vi "HEWH HeatUp Test Selector.vi"(4 "Standard Heat-Up (80 Gallon) Heat Pump":T1[](array[typedef]) {"Time" format="%<%H:%M:%S>t"}, 6 "Standard Heat-Up (80 Gallon)":T1[](array[typedef]) {"Time" format="%<%H:%M:%S>t"}, 7 "Standard Heat-Up (50 Gallon) Heat Pump in":T1[](array[typedef]) {"Time" format="%<%H:%M:%S>t"}, 8 "Error In":errorcluster, 9 "Heating Mode":string, 10 "Unit Type":T8, 11 "Standard Heat-Up (50 Gallon)":T1[](array[typedef]) {"Time" format="%<%H:%M:%S>t"}) -> (0 "Error Out":errorcluster, 3 "Standard Heat-Up (50 Gallon) Heat Pump out":T1[](array[typedef]) {"Time" format="%<%H:%M:%S>t"})   [LabVIEW 2016]
uses:
  Type Definitions/PRAT Test.ctl
  Utility/Save File/File Setup (Public)/Type Definition/Save File HEWH Heating Control Mode.ctl
  Draw Water Specific/Type Definitions/Terminate Draw Conditions.ctl
  Type Definitions/HEWH Start Conditions.ctl
  Draw Water Specific/Type Definitions/Check Special Condtions.ctl
  Draw Water Specific/Type Definitions/HEWH Special Condition Check.ctl
  Type Definitions/HEWH Draw Flag ENUM.ctl
  Draw Water Specific/Type Definitions/Unit Type.ctl
  Utility/Save File/File Setup.lvlib
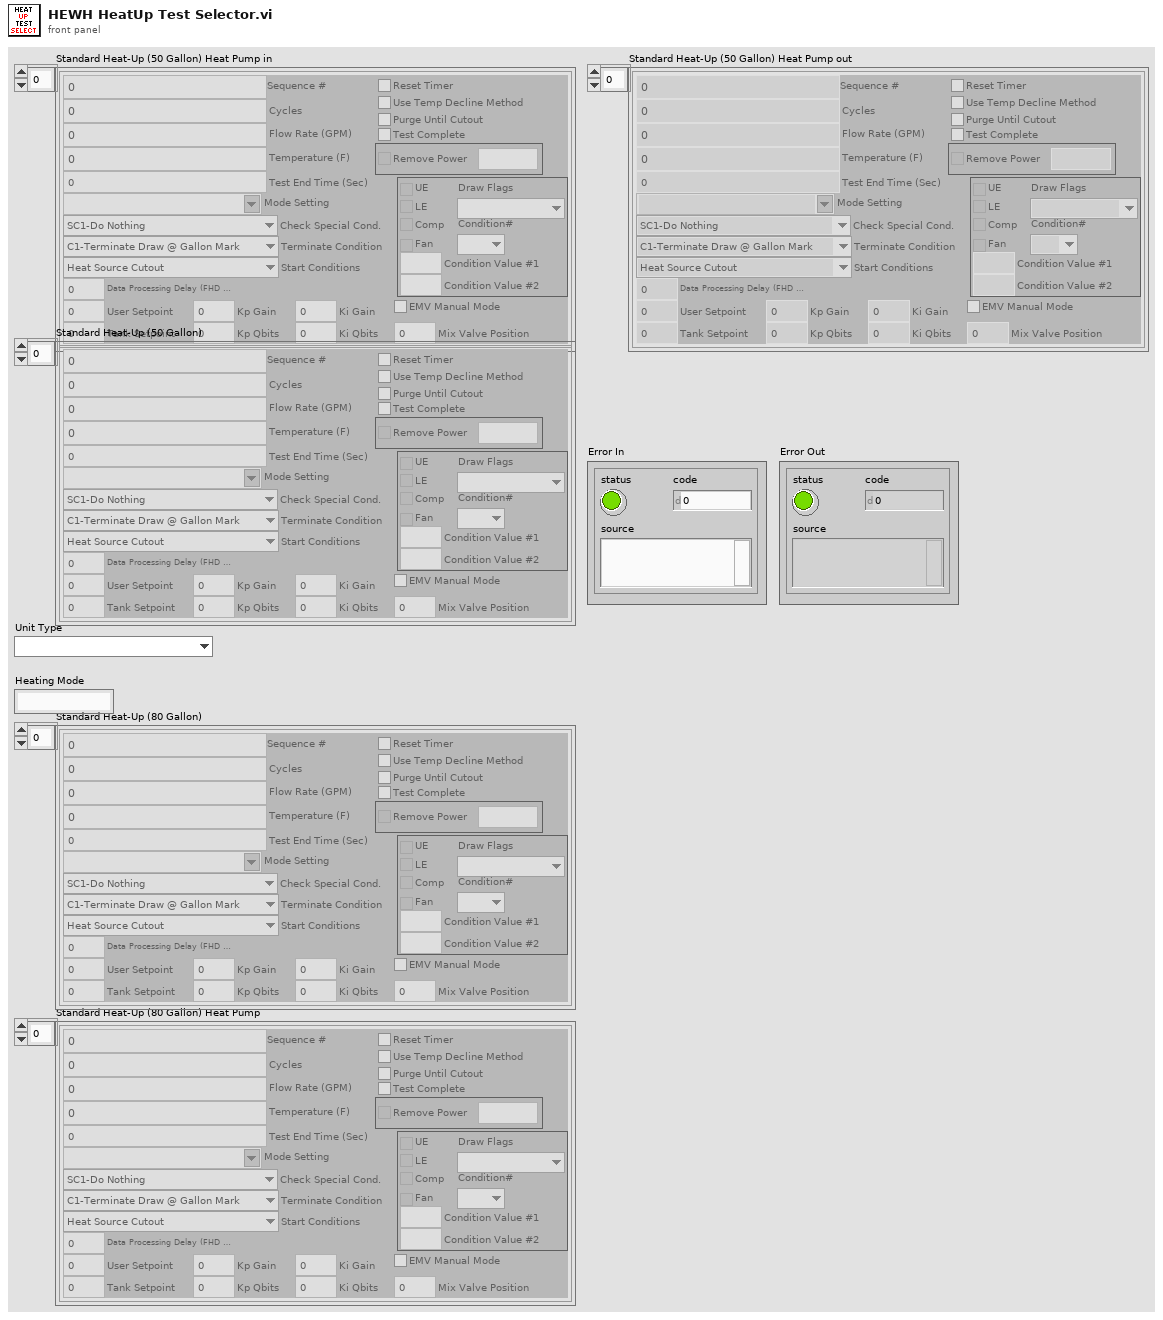
[diagram p1: front panel]
types:
  T1 = typedef "PRAT Test.ctl" = cluster{"Sequence #":dbl, "Cycles":i32, "Mode Setting":T2, "Flow Rate (GPM)":dbl, "Temperature (F)":dbl, "Reset Timer":bool, "Use Temp Decline Method":bool, "Terminate Condition":T3, "Condition Value #1":dbl, "UE":bool, "LE":bool, "Comp":bool, "Fan":bool, "Test End Time (Sec)":dbl, "Purge Until Cutout":bool, "Start Conditions":T4, "Condition Value #2":dbl, "Remove Power":bool, "Time":dbl, "Check Special Cond.":T5, "Condition#":T6, "Draw Flags":T7, "Data Processing Delay (FHD 15sec, UEF 5 Sec)":dbl, "Test Complete":bool, "User Setpoint":dbl, "Tank Setpoint":dbl, "Kp Gain":dbl, "Kp Qbits":dbl, "Ki Gain":dbl, "Ki Qbits":dbl, "Mix Valve Position":i16, "EMV Manual Mode":bool}
  T2 = typedef "File Setup.lvlib/Save File HEWH Heating Control Mode.ctl" = string
  T3 = typedef "Terminate Draw Conditions.ctl" = enum16{"C1-Terminate Draw @ Gallon Mark", "C2-Special Last Draw (HU Test)", "C3-RTD Out <=", "C4-Mean Tank Temp <=", "C5-Decrease RTD Out (Deg F)", "C6-Time (Seconds)", "C7-Until Any Heat Source", "C8-Specific Heat Source", "C9-Do Nothing"}
  T4 = typedef "HEWH Start Conditions.ctl" = enum16{"Heat Source Cutout", "At Time (Seconds)", "Every X (Seconds)", "T2 >= X° Below Setpoint", "Seconds From Complete", "Wait for LE & Comp Cutout", "Wait for Comp Cutout", "Wait for LE Cutout", "Wait for UE Cutout"}
  T5 = typedef "Check Special Condtions.ctl" = enum16{"SC1-Do Nothing", "SC2-Check Heat Source (On-C2/Off-C1)", "SC3-Check Skip Condition", "SC4-Check Heat Source ON/Fail"}
  T6 = typedef "HEWH Special Condition Check.ctl" = enum16{"N/A", "C1", "C2", "Reset/Fail", "Skip Draw Sequence"}
  T7 = typedef "HEWH Draw Flag ENUM.ctl" = enum16{"N/A", "None(0)", "Sml(1)", "Med(2)", "SmlMed(3)", "Lrg(4)", "SmlLrg(5)", "MedLrg(6)", "SmlMedLrg(7)"}
  T8 = typedef "Unit Type.ctl" = enum16{"", "50 Gallon", "80 Gallon"}
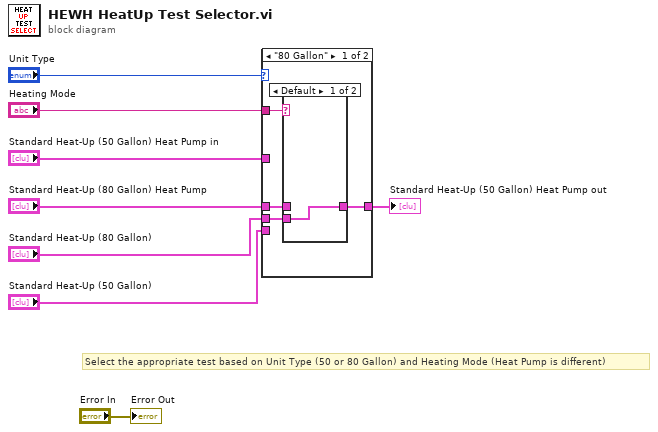
[diagram p0: block diagram]
diagram:
  # "Select the appropriate test based on Unit Type (50 or 80 Gallon) and Heating Mode (Heat Pump is different)"
  n1 = case shown="\"80 Gallon\"" "Unit Type" {
    tunnel: [w12 w18] -> w2
    tunnel: "Heating Mode" -> [w11 w17]
    tunnel: "Standard Heat-Up (80 Gallon)" -> [w10 _]
    tunnel: "Standard Heat-Up (80 Gallon) Heat Pump" -> [w9 _]
    tunnel: "Standard Heat-Up (50 Gallon)" -> [_ w16]
    tunnel: "Standard Heat-Up (50 Gallon) Heat Pump in" -> [_ w15]
    frame "80 Gallon" {
      n2 = case shown="Default" w11 {
        tunnel: [w13 w14] -> w12
        tunnel: w10 -> [w13 _]
        tunnel: w9 -> [_ w14]
        frame Default {
        }
        frame "Heat Pump" {
        }
      }
    }
    frame "50 Gallon", Default {
      n3 = case shown="\"Heat Pump\"" w17 {
        tunnel: [w19 w20] -> w18
        tunnel: w16 -> [w19 _]
        tunnel: w15 -> [_ w20]
        frame Default {
        }
        frame "Heat Pump" {
        }
      }
    }
  }
  "Standard Heat-Up (50 Gallon) Heat Pump out" <- w2
  "Error Out" <- "Error In"
